vi "runViAnalyzer.vi"() -> ()   [LabVIEW 2023]
doc: "This example uses the advanced VI Analyzer VIs to perform an analysis on an LLB of VIs. The \"New Task\" VI uses preset test settings loaded from a CFG file that was created from the VI Analyzer user interface. Certain advanced VIs are used to perform tasks like adding an LLB to the analysis, removing a single VI from the analysis, removing certain tests from the analysis, and modifying a configuration value on one test. Once the analysis performed by \"VIAn Run.vi\" is complete, the \"VIAn Easy Report.vi\" saves the analysis results to an HTML report."
uses:
  <vilib>/addons/analyzer/NI_VIAnalyzerTKVIs.lvlib
  <vilib>/Wiresmith Technology/G CLI/CLI Class/CLI.lvclass
panel:
  out "Custom Parameters":string[](array[string])
  out "VI in Analysis":string
  out "Analysis Progress":dbl(slide) scale=0.0..100.0
  out "Tests Run":string[](array[string])
  out "VIs Tested":path[](array[path])
  # "Overview: Demonstrates the use of the VI Analyzer and VI Analyzer Utility VIs to customize a programmatic analysis.\nRequirements: VI Analyzer Toolkit\nInstructions:\nRun the VI."
  # "Exclude these tests from the VI Analyzer Task."
  # "Set these tests to have 10 maximum failures for the VI Analyzer Task."
  # "Remove the top-level placeholder VI from the analysis."
  # "Disable the option on the \"VI Documentation\" test to analyze control descriptions."
  # "Show the progress of the analysis."
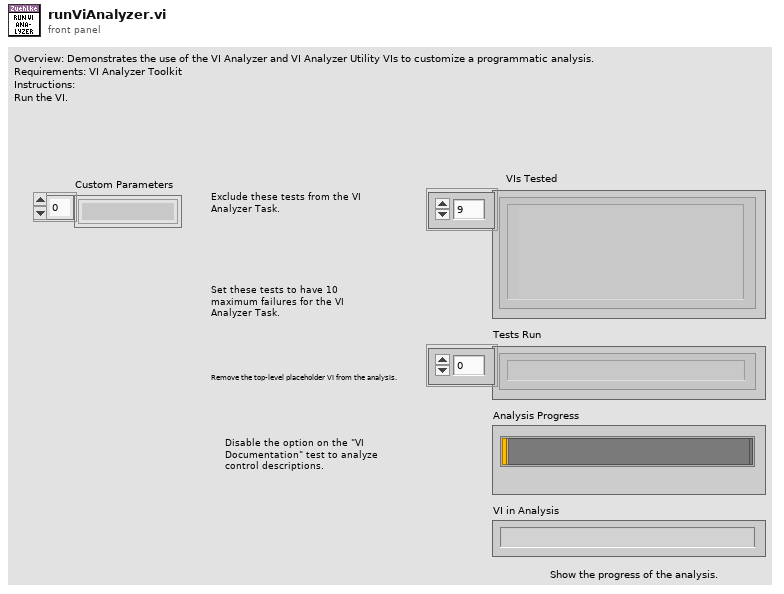
[diagram p1: front panel]
types:
  T1 = typedef "VIAnAPI Ref.ctl" = refnum<k1>
  T2 = typedef "VIAnCtl Results.ctl" = cluster{"Test Name":string, "Results Data":T3[], "Status":T4, "Exceed Max Fails?":bool}
  T3 = typedef "VIAnCtl ResultsData (index).ctl" = cluster{"Result Message":string, "Ref Index":i32}
  T4 = typedef "VIAnCtl ResultStatus.ctl" = enum16{"Pass", "Fail", "Skipped", "VI not loadable", "Test not loadable", "Test not runnable", "Test error out"}
  T5 = typedef "VIAnRes Parsed Results Data (by VI).ctl" = cluster{"VI Path":path, "Pass":cluster{"row":i32, "column":i32}[], "Fail":cluster{"row":i32, "column":i32}[], "Skipped":cluster{"row":i32, "column":i32}[], "VI not loadable":cluster{"row":i32, "column":i32}[], "Test not loadable":cluster{"row":i32, "column":i32}[], "Test not runnable":cluster{"row":i32, "column":i32}[], "Test error out":cluster{"row":i32, "column":i32}[]}
  T6 = typedef "VIAnRes Parsed Results Data (by Test).ctl" = cluster{"Test Name":string, "Pass":cluster{"VI Path":path, "index":cluster{"row":i32, "column":i32}}[], "Fail":cluster{"VI Path":path, "index":cluster{"row":i32, "column":i32}}[], "Skipped":cluster{"VI Path":path, "index":cluster{"row":i32, "column":i32}}[]}
  T7 = typedef "VIAnCtl Test Config Data.ctl" = cluster{"Test Name":string, "Config Ref":refnum<vi>, "Ref Valid?":bool, "Test Ranking":T8, "Max Failures":u32, "Test Path":path, "Control Values":T9[], "Selected?":bool}
  T8 = typedef "VIAnCtl TestRanking.ctl" = u16
  T9 = typedef "VIAnCtl Config Control Value.ctl" = cluster{"Control Name":string, "Control Value":variant}
  T10 = cluster{"Raw Results":T2[][], "Parsed Results Data (by VI)":T5[], "Parsed Results Data (by Test)":T6[], "Summary Statistics":cluster{"Passed Tests":i32, "Failed Tests":i32, "Skipped Tests":i32, "VIs not loadable":i32, "Tests not loadable":i32, "Tests not runnable":i32, "Test error out":i32, "Start Time":u32, "Total Time (s)":dbl}, "Test Config Data":T7[]}
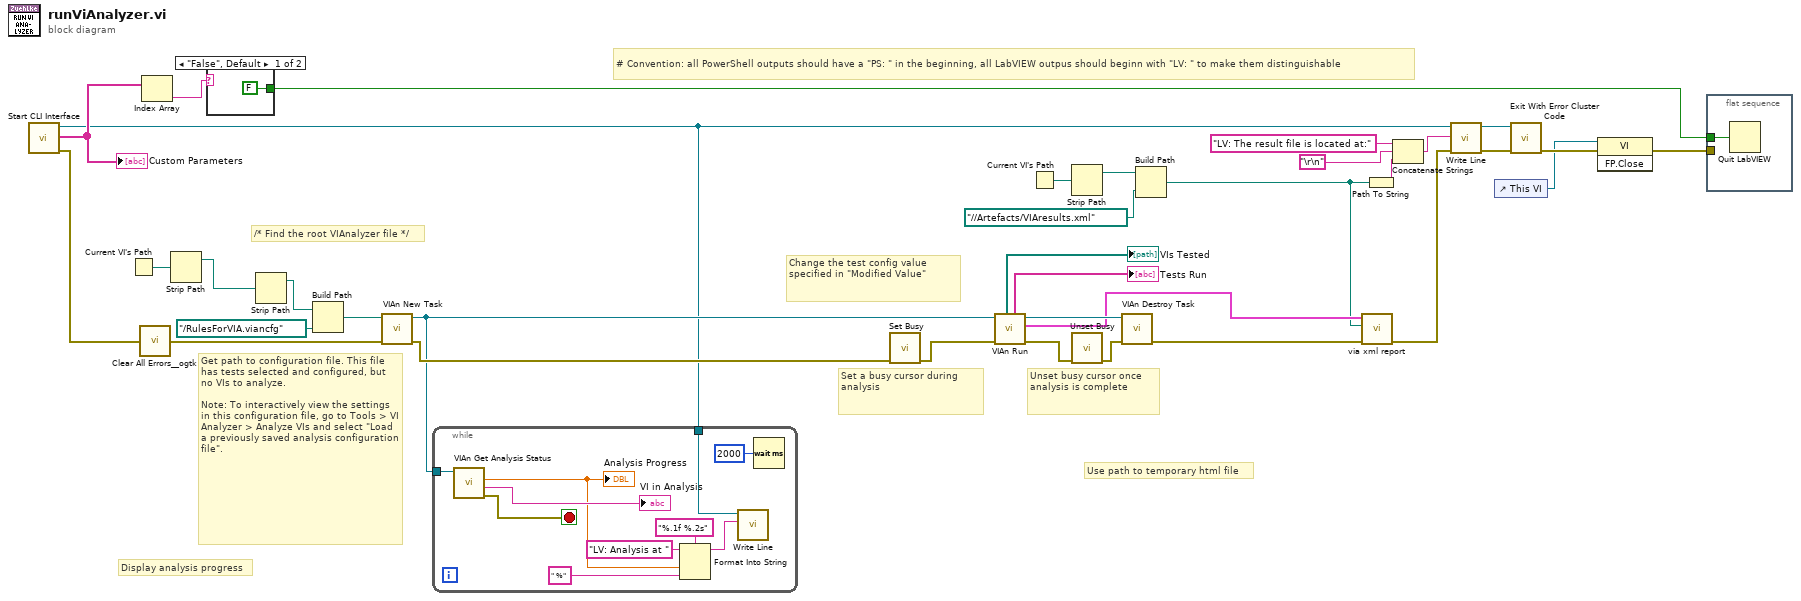
[diagram p0: block diagram]
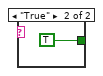
[diagram p2: hidden frame]
diagram:
  # "# Convention: all PowerShell outputs should have a \"PS: \" in the beginning, all LabVIEW outpus should beginn with \"LV: \" to make them distinguishable"
  # "/* Find the root VIAnalyzer file */"
  # "Display analysis progress"
  # "Unset busy cursor once analysis is complete"
  # "Set a busy cursor during analysis"
  # "Use path to temporary html file"
  # "Change the test config value specified in \"Modified Value\""
  # "Get path to configuration file. This file has tests selected and configured, but no VIs to analyze.\n\nNote: To interactively view the settings in this configuration file, go to Tools > VI Analyzer > Analyze VIs and select \"Load a previously saved analysis configuration file\"."
  n1 = call <vilib>:"Start CLI Interface.vi"() -> ("error out"=w19:errorcluster, "Custom Parameters"=w18:string[], "CLI out"=w15:refnum<class "CLI.lvclass">)  [unwired: 8 in, 1 out]
  "Custom Parameters" <- w18
  n2 = Current VI's Path() -> (path=w26:path)
  n3 = call <userlib>:"Clear All Errors__ogtk.vi"("Error In"=w19) -> ("Error Out"=w6:errorcluster)  [unwired: 3 in]
  n4 = Index Array(array=w18) -> (element=w17:string)  [unwired: 1 in]
  n5 = Strip Path(path=w26) -> (stripped path=w2:path)  [unwired: 1 out]
  n6 = case shown="\"False\", Default" w17 {
    tunnel: [FALSE TRUE] -> w16
    frame "False", Default {
    }
    frame "True" {
    }
  }
  n7 = Strip Path(path=w2) -> (stripped path=w1:path)  [unwired: 1 out]
  n8 = Build Path(base path=w1, name or relative path=path "../RulesForVIA.viancfg" ("path")) -> (appended path=w25:path)
  n9 = call <vilib>:"VIAn New Task.vi"("error in (no error)"=w6, "Path to Configuration File"=w25) -> ("error out"=w35:errorcluster, "VI Analyzer Task"=w28:T1)  [unwired: 1 in, 7 out]
  n10 = while {
    tunnel: w28 -> [w47]
    tunnel: w15 -> [w43]
    stop <- w44 stop-if-true
    n11 = call <vilib>:"VIAn Get Analysis Status.vi"("VI Analyzer Task in"=w47) -> ("error out"=w44:errorcluster, "VI in Analysis"=→"VI in Analysis":string, "Percent Complete"=w42:dbl)  [unwired: 1 in, 7 out]
    "Analysis Progress" <- w42
    n12 = Format Into String(format string="%.1f %.2s", initial string="LV: Analysis at ", w42, " %" ("initial string")) -> (resulting string=w39:string)  [unwired: 1 in, 1 out]
    n13 = call <vilib>:"Write Line.vi"("Text to Write"=w39, "CLI in"=w43) -> ()  [unwired: 8 in, 2 out]
    n14 = Wait (ms)(milliseconds to wait=u32 2000) -> ()  [unwired: 1 out]
  }
  n15 = call <vilib>:"Set Busy.vi"("error in (no error)"=w35) -> ("error out"=w31:errorcluster)  [unwired: 3 in, 7 out]
  n16 = call <vilib>:"VIAn Run.vi"("error in (no error)"=w31, "VI Analyzer Task in"=w28) -> ("error out"=w30:errorcluster, "Analysis Results"=w20:T10, "VI Analyzer Task out"=w34:T1, "Tests Run"=→"Tests Run":string[], "VIs Tested"=→"VIs Tested":path[])  [unwired: 5 out]
  n17 = Current VI's Path() -> (path=w23:path)
  n18 = Strip Path(path=w23) -> (stripped path=w24:path)  [unwired: 1 out]
  n19 = call <vilib>:"Unset Busy.vi"("error in (no error)"=w30) -> ("error out"=w29:errorcluster)  [unwired: 1 in, 9 out]
  n20 = call <vilib>:"VIAn Destroy Task.vi"("error in (no error)"=w29, "VI Analyzer Task in"=w34) -> ("error out"=w21:errorcluster)  [unwired: 9 out]
  n21 = Build Path(base path=w24, name or relative path=path "../../Artefacts/VIAresults.xml" ("path")) -> (appended path=w9:path)
  n22 = call <vilib>:"via xml report.vi"("error in (no error)"=w21, "Path"=w9, "Analysis Results"=w20) -> ("error out"=w13:errorcluster)  [unwired: 8 in]
  n23 = Path To String(path=w9) -> (string=w10:string)
  n24 = Concatenate Strings("LV: The result file is located at:" ("string"), "\r\n", w10) -> (w8:string)
  n25 = call <vilib>:"Write Line.vi"("error in (no error)"=w13, "Text to Write"=w8, "CLI in"=w15) -> ("error out"=w7:errorcluster, "CLI out"=w14:refnum<class "CLI.lvclass">)  [unwired: 7 in]
  n26 = control-ref of="This VI"() -> (w3:refnum<vi>)
  n27 = call <vilib>:"Exit With Error Cluster Code.vi"("error in (no error)"=w7, "CLI in"=w14) -> ("error out"=w5:errorcluster)  [unwired: 9 in]
  n28 = invoke class="VI" method="FP.Close"(reference=w3, error in=w5) -> (error out=w4:errorcluster)  [unwired: 1 in, 2 out]
  n29 = flat-sequence {
    tunnel: w4 -> [_]
    tunnel: w16 -> [w48]
    frame #0 {
      n30 = Quit LabVIEW(quit? (T)=w48) -> ()
    }
  }
